vi "set_amplitudes.vi"(8 "error in (no error)":errorcluster, 9 "y amplitude":dbl[unit], 10 "x amplitude":dbl[unit], 11 "TrajectoryTS090820Circular2D in":refnum<class "TrajectoryTS090820Circular2D.lvclass">) -> (0 "error out":errorcluster, 3 "TrajectoryTS090820Circular2D out":refnum<class "TrajectoryTS090820Circular2D.lvclass">)   [LabVIEW 2010, in "TrajectoryTS090820Circular2D.lvclass"]
uses:
  TrajectoryTS090820Circular2D.lvclass
  TrajectoryTS090820Circular2D.lvclass/TrajectoryTS090820Circular2D.ctl
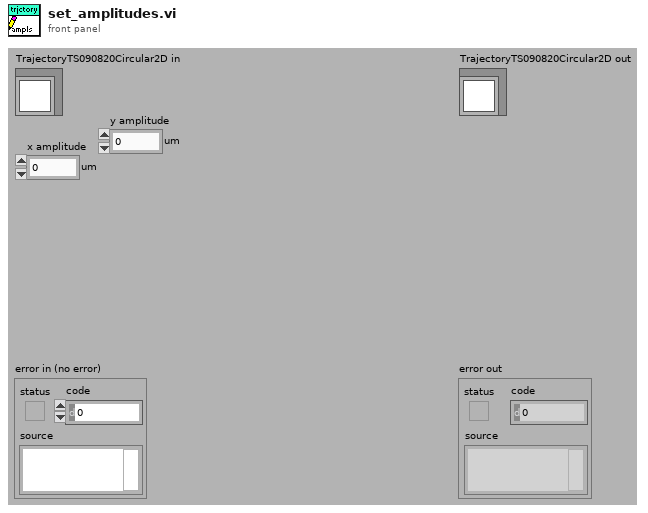
[diagram p1: front panel]
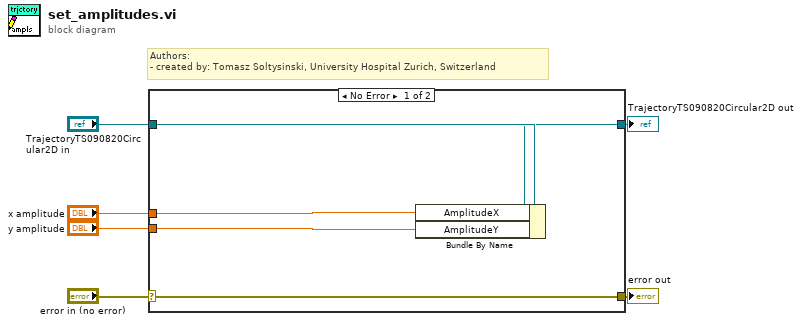
[diagram p0: block diagram]
diagram:
  # "Authors: \n- created by: Tomasz Soltysinski, University Hospital Zurich, Switzerland"
  n1 = case shown="No Error" "error in (no error)" {
    selector: "error in (no error)" -> [w11 w12]
    tunnel: [w11 w12] -> w5
    tunnel: [w9 w13] -> w3
    tunnel: "TrajectoryTS090820Circular2D in" -> [w10 w13]
    tunnel: "x amplitude" -> [w8 _]
    tunnel: "y amplitude" -> [w7 _]
    frame No Error {
      n2 = Bundle By Name(cluster=w10, "AmplitudeX"=w8, "AmplitudeY"=w7) -> (w9:refnum<class "TrajectoryTS090820Circular2D.lvclass">)
    }
    frame Error {
    }
  }
  "error out" <- w5
  "TrajectoryTS090820Circular2D out" <- w3
